vi "Shoot.vi"(2 "Shoot":bool=TRUE) -> ()   [LabVIEW 2016]
uses:
  <vilib>/Rock Robotics/WPI/SafetyOutput/WPI_SafetyOutputConfigMenu.ctl
  Global 2.vi
  <vilib>/gmath/NI_Gmath.lvlib
panel:
  in  "Adjustment X":dbl[](array[numeric])=[-3400.0, -3100.0, -2750.0, -2430.0, -2080.0, -1710.0, -1330.0, -950.0, -580.0, -210.0, 0.0, 210.0, 580.0, 950.0, 1330.0, 1710.0, 2080.0, 2430.0, 2750.0, 3100.0, 3400.0]
  in  "Adjustment Y":dbl[](array[numeric])=[-1.0, -0.9, -0.8, -0.7, -0.6, -0.5, -0.4, -0.3, -0.2, -0.1, 0.0, 0.1, 0.2, 0.3, 0.4, 0.5, 0.6, 0.7, 0.8, 0.9, 1.0] format="%_6g"
  out "Waveform Chart":cluster{dbl}(graph)={2565.46875}
  out "Motor Effort":dbl=0.17108041660508766
  out "Adjustment":dbl=-0.27365642550017555
  out "RPM":dbl=2565.46875
  in  "kP":dbl=0.8 format="%#_13g"
  in  "kD":dbl=0.06 format="%#_13g"
  in  "Y":dbl[](array[numeric])=[0.0, 0.1, 0.2, 0.3, 0.4, 0.5, 0.6, 0.7, 0.8, 0.9, 1.0] format="%_6g"
  in  "X":dbl[](array[numeric])=[0.0, 210.0, 580.0, 950.0, 1330.0, 1710.0, 2080.0, 2430.0, 2750.0, 3100.0, 3400.0]
  in  "RPM Target BB":dbl=1500.0
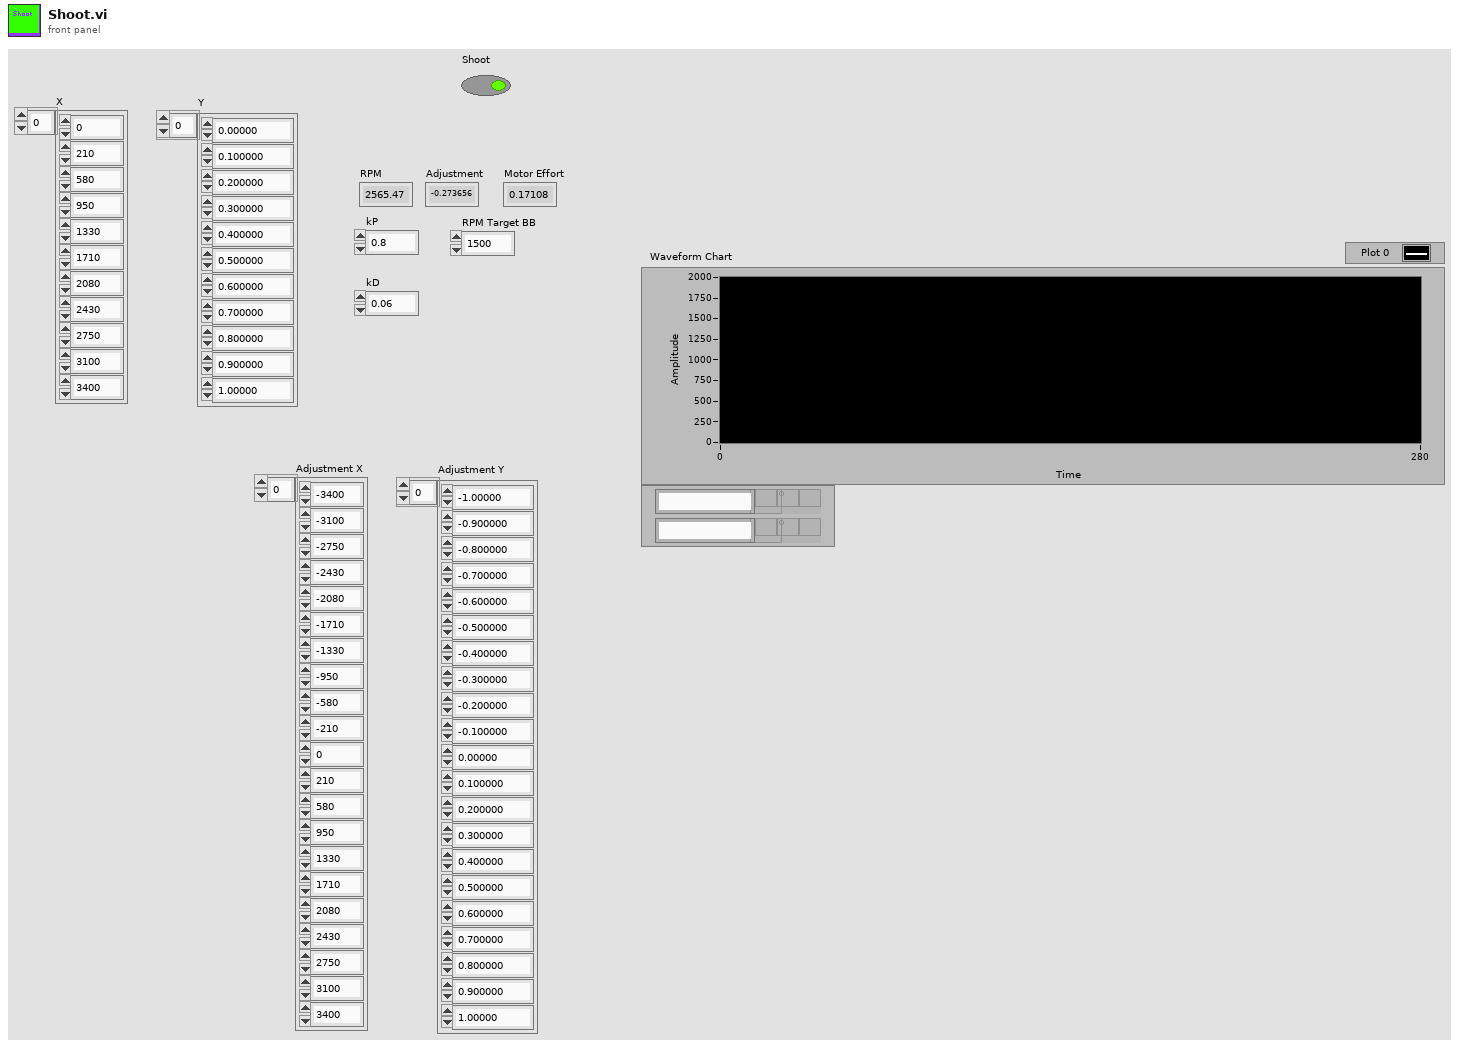
[diagram p1: front panel]
types:
  T1 = typedef "WPI_SafetyOutputConfigMenu.ctl" = enum16{"Enable", "Disable"}
  T2 = typedef "WPI_MotorControlDeviceRef.ctl" = cluster{"DeviceStatus":errorcluster, "Type":T3, "PWM":cluster{"PWM Channel":T4, "DeadBand":T5}, "CAN":cluster{"Device Number":u8, "SetOutput VI Ref":variant, "GetOutput VI Ref":variant, "Enable VI Ref":variant, "Disable VI Ref":variant, "Data":variant}, "Invert":bool}
  T3 = typedef "WPI_MotorControlType.ctl" = enum16{"PWM", "CAN"}
  T4 = typedef "FPGA_DIOPWMChannel.ctl" = enum8{"PWM 0", "PWM 1", "PWM 2", "PWM 3", "PWM 4", "PWM 5", "PWM 6", "PWM 7", "PWM 8", "PWM 9", "PWM MXP 0", "PWM MXP 1", "PWM MXP 2", "PWM MXP 3", "PWM MXP 4", "PWM MXP 5", "PWM MXP 6", "PWM MXP 7", "PWM MXP 8", "PWM MXP 9", "Invalid"}
  T5 = typedef "WPI_PWMDeadband.ctl" = cluster{"Name":string, "maxPositivePwm":i32, "minPositivePwm":i32, "centerPwm":i32, "maxNegativePwm":i32, "minNegativePwm":i32, "angularRange":u16}
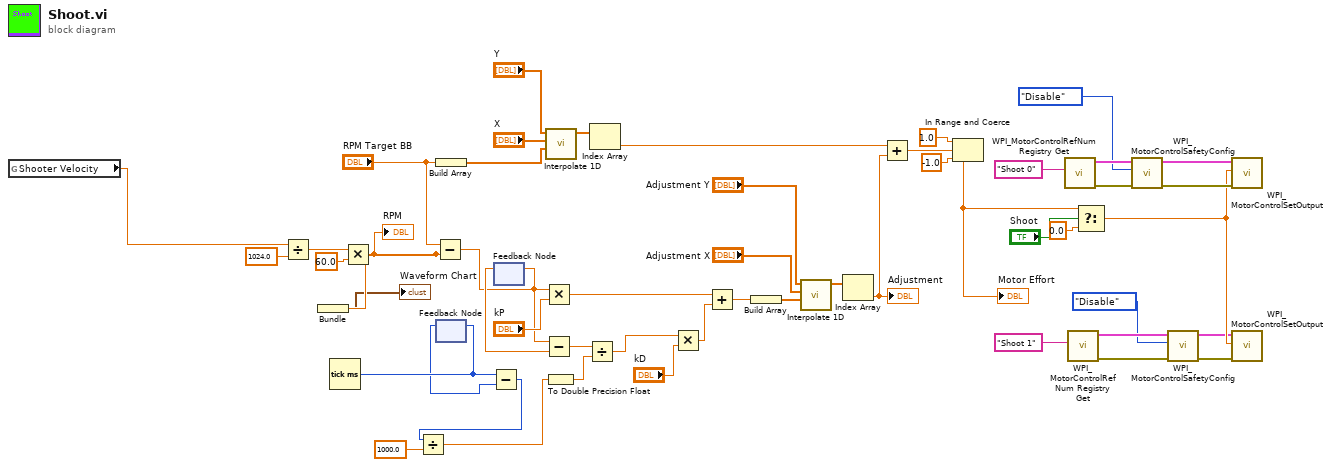
[diagram p0: block diagram]
diagram:
  n1 = global read "Global 2.vi" "Shooter Velocity"() -> (w15:dbl)
  n2 = Divide(x=w15, y=1024.0) -> (x/y=w49:dbl)
  n3 = Tick Count (ms)() -> (millisecond timer value=w44:u32)
  n4 = Multiply(x=w49, y=60.0) -> (x*y=w21:dbl)
  "RPM" <- w21
  n5 = Bundle(w21) -> (→"Waveform Chart":cluster{dbl})  [unwired: 1 in]
  n6 = Subtract(x="RPM Target BB", y=w21) -> (x-y=w23:dbl)
  n7 = Build Array("RPM Target BB") -> (w47:dbl[])
  n8 = feedback #1() -> (w43:u32)  [unwired: 1 in]
  n9 = feedback-in #1(w44) -> ()
  n10 = Subtract(x=w44, y=w43) -> (x-y=w2:u32)
  n11 = Divide(x=w2, y=1000.0) -> (x/y=w1:dbl)
  n12 = feedback #2() -> (w45:dbl)  [unwired: 1 in]
  n13 = feedback-in #2(w23) -> ()
  n14 = Multiply(x=w23, y="kP") -> (x*y=w36:dbl)
  n15 = Subtract(x=w23, y=w45) -> (x-y=w42:dbl)
  n16 = call <vilib>:"Interpolate 1D.vi"("xi"=w47, "X"="X", "Y"="Y") -> ("yi"=w46:dbl[])  [unwired: 6 in, 2 out]
  n17 = To Double Precision Float(number=w1) -> (double precision float=w41:dbl)
  n18 = Divide(x=w42, y=w41) -> (x/y=w40:dbl)
  n19 = Index Array(array=w46) -> (element=w34:dbl)  [unwired: 1 in]
  n20 = Multiply(x=w40, y="kD") -> (x*y=w35:dbl)
  n21 = Add(x=w36, y=w35) -> (x+y=w29:dbl)
  n22 = Build Array(w29) -> (w32:dbl[])
  n23 = call <vilib>:"Interpolate 1D.vi"("xi"=w32, "X"="Adjustment X", "Y"="Adjustment Y") -> ("yi"=w33:dbl[])  [unwired: 6 in, 2 out]
  n24 = Index Array(array=w33) -> (element=w28:dbl)  [unwired: 1 in]
  "Adjustment" <- w28
  n25 = Add(x=w34, y=w28) -> (x+y=w27:dbl)
  n26 = In Range and Coerce(upper limit=1.0, x=w27, lower limit=-1.0 ("upper limit")) -> (coerced(x)=w24:dbl)  [unwired: 1 out]
  "Motor Effort" <- w24
  n27 = call <vilib>:"WPI_MotorControlRefNum Registry Get.vi"("refnum name"="Shoot 0") -> ("error out"=w4:errorcluster, "MotorControlDevRef"=w14:T2)  [unwired: 9 in]
  n28 = call <vilib>:"WPI_MotorControlRefNum Registry Get.vi"("refnum name"="Shoot 1") -> ("error out"=w9:errorcluster, "MotorControlDevRef"=w10:T2)  [unwired: 9 in]
  n29 = Select(t=w24, s="Shoot", f=0.0) -> (s? t:f=w8:dbl)
  n30 = call <vilib>:"WPI_MotorControlSafetyConfig.vi"("error in (no error)"=w4, "mode"=WPI_SafetyOutputConfigMenu."Disable", "MotorControlDevRef"=w14) -> ("error out"=w12:errorcluster, "MotorControlDevRef"=w13:T2)  [unwired: 7 in]
  n31 = call <vilib>:"WPI_MotorControlSafetyConfig.vi"("error in (no error)"=w9, "mode"=WPI_SafetyOutputConfigMenu."Disable", "MotorControlDevRef"=w10) -> ("error out"=w6:errorcluster, "MotorControlDevRef"=w7:T2)  [unwired: 7 in]
  n32 = call <vilib>:"WPI_MotorControlSetOutput.vi"("error in (no error)"=w12, "Output"=w8, "MotorControlDevRef"=w13) -> ()  [unwired: 6 in, 3 out]
  n33 = call <vilib>:"WPI_MotorControlSetOutput.vi"("error in (no error)"=w6, "Output"=w8, "MotorControlDevRef"=w7) -> ()  [unwired: 6 in, 3 out]
